vi "Owl429_TxAcyclicTransferConfig_getLabel.vi"(8 "error in (no error)":errorcluster, 11 "acyclic config handle":u32) -> (0 "error out":errorcluster, 2 "label":u8, 3 "acyclic config handle":u32)   [LabVIEW 2012, in "AIT 429 System Explorer.lvlib"]
doc: "Gets the value of the label field for the label transfer.\n\nReturns:\nThe label value."
uses:
  AIT 429 System Explorer.lvlib
  <userlib>/ARINC-429/Owl429.lvlib
  owl429.dll
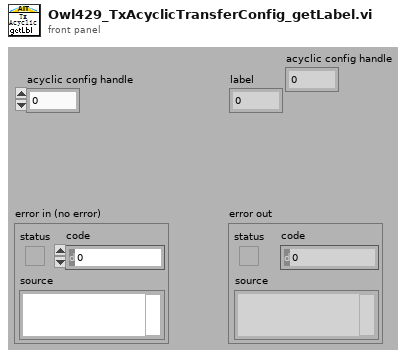
[diagram p1: front panel]
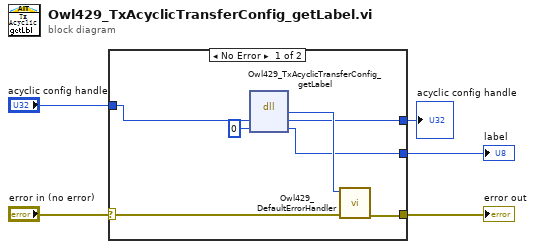
[diagram p0: block diagram]
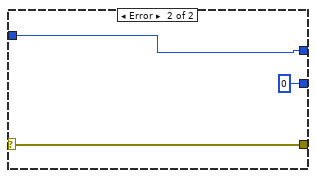
[diagram p2: hidden frame]
diagram:
  n1 = case shown="No Error" "error in (no error)" {
    selector: "error in (no error)" -> [w9 w15]
    tunnel: [w8 w15] -> w4
    tunnel: "acyclic config handle" -> [w11 w14]
    tunnel: [w10 u8 0 ("label")] -> w2
    tunnel: [w6 w14] -> w1
    frame No Error {
      n2 = dll-call lib="owl429.*" fn="Owl429_TxAcyclicTransferConfig_getLabel" ("429owl.*:Owl429_TxScheduledLabelConfig_getLabel")("label config handle"=w11, "label"=u8 0) -> ("return type"=w12:i32, "label config handle"=w6:u32, "label"=w10:u8)  [unwired: 3 in, 2 out]
      n3 = call <userlib>:"Owl429_DefaultErrorHandler.vi"("error in (no error)"=w9, "error code"=w12) -> ("error out"=w8:errorcluster)  [unwired: 9 in]
    }
    frame Error {
    }
  }
  "label" <- w2
  "error out" <- w4
  "acyclic config handle" <- w1
